vi "Week2_Slide19_ResetCounterLogic.vi"() -> ()   [LabVIEW 2015]
panel:
  in  "Reset":bool
  out "Counter":dbl
  in  "stop":bool
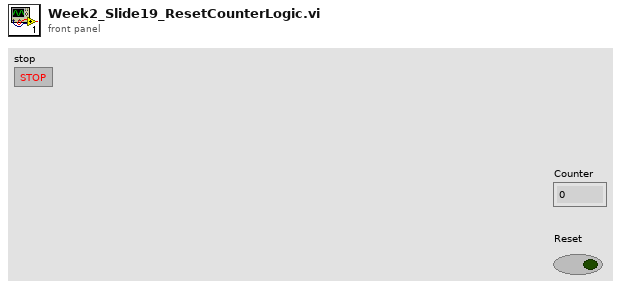
[diagram p1: front panel]
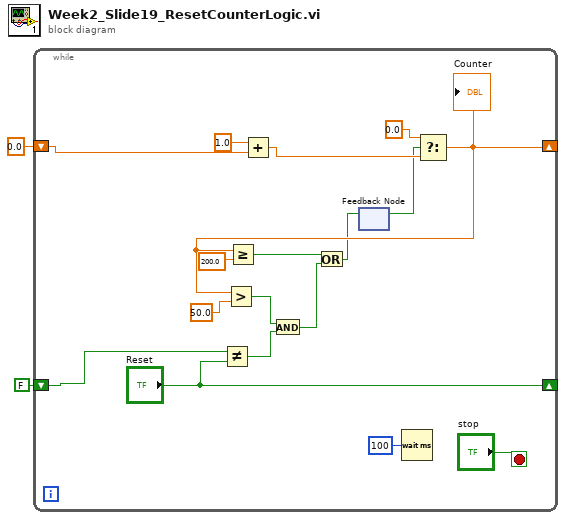
[diagram p0: block diagram]
diagram:
  n1 = while {
    shift-right: [w8] -> _
    shift-left: 0.0 -> [w17]
    shift-right: ["Reset"] -> _
    shift-left: FALSE ("Reset") -> [w14]
    stop <- "stop" stop-if-true
    n2 = Not Equal?(x=w14, y="Reset") -> (x != y?=w9:bool)
    n3 = Add(x=1.0, y=w17) -> (x+y=w13:dbl)
    n4 = feedback #1() -> (w3:bool)  [unwired: 1 in]
    n5 = Wait (ms)(milliseconds to wait=u32 100) -> ()  [unwired: 1 out]
    n6 = Select(t=0.0 ("f"), s=w3, f=w13) -> (s? t:f=w8:dbl)
    "Counter" <- w8
    n7 = Greater?(x=w8, y=50.0) -> (0:w10:bool)
    n8 = Greater Or Equal?(x=w8, y=200.0) -> (x >= y?=w6:bool)
    n9 = And(x=w10, y=w9) -> (x .and. y?=w5:bool)
    n10 = Or(x=w6, y=w5) -> (x .or. y?=w4:bool)
    n11 = feedback-in #1(w4) -> ()
  }
